vi "ChangeInheritance.vi"(0 "ClassWriterGOOP300 in":refnum<class "ClassWriterGOOP400.lvclass">, 1 "LvClass":refnum<vi>, 2 "NewBaseClass(Empty=ConvertClassToBaseClass)":path=path "C:/Documents and Settings/Micke/Skrivbord/My Computer/B_class/B.lvclass", 5 "error in (no error)":errorcluster) -> (14 "ClassWriterGOOP300 out":refnum<class "ClassWriterGOOP400.lvclass">, 19 "error out":errorcluster)   [LabVIEW 2020, in "ClassWriterGOOP400.lvclass"]
uses:
  <resource>/Framework/Providers/Open_GDS/ClassProviders/Provider_EndevoGOOP400/ClassWriterGOOP400_class/ClassWriterGOOP400.lvclass
  <resource>/Framework/Providers/Open_GDS/ClassProviders/Provider_EndevoGOOP400/Templates/EndevoG4TemplateNames.ctl
  <resource>/Framework/Providers/Open_GDS/ClassProviders/Provider_LvNativeClass/ClassWriterNative_class/ClassWriterNative.lvclass
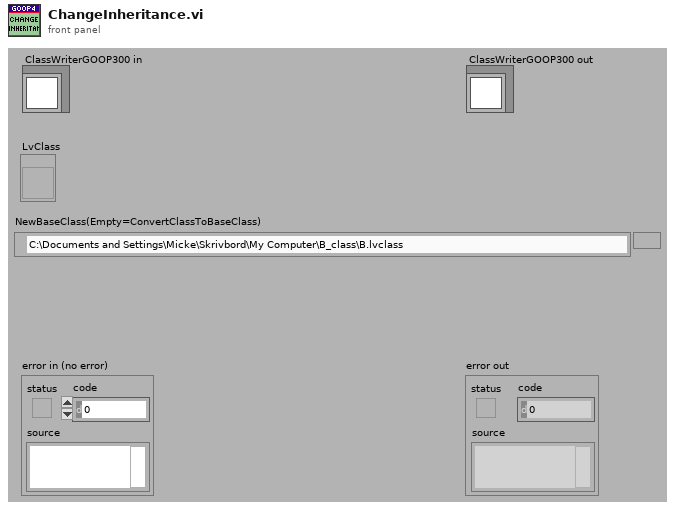
[diagram p1: front panel]
types:
  T1 = typedef "EndevoG4TemplateNames.ctl" = enum16{"G4BaseTemplate_Simple_4x4x4", "G4SubTemplate_Simple_4x4x4", "G4BaseTemplate_Simple_6x8x6", "G4SubTemplate_Simple_6x8x6", "G4BaseTemplate_Singleton_4x4x4", "G4SubTemplate_Singleton_4x4x4", "G4BaseTemplate_Singleton_6x8x6", "G4SubTemplate_Singleton_6x8x6", "G4InterfaceTemplate_6x8x6", "G4InterfaceTemplate_4x4x4", "G4BaseTemplate_Simple_5x6x5", "G4BaseTemplate_Singleton_5x6x5", "G4InterfaceTemplate_5x6x5", "G4SubTemplate_Simple_5x6x5", "G4SubTemplate_Singleton_5x6x5"}
  T2 = typedef "GDSLvCLass_ClassSettingsType.ctl" = cluster{"ClassProviderName":string, "ClassTemplateUsed":string, "ClassTemplateVersion":string, "ClassDescription":string, "PlugIns":T3[], "ConnectorPanePattern":string}
  T3 = typedef "GDSLvClass_PlugIn.ctl" = cluster{"Type":T4, "ID":string, "Version":string, "Path":path, "Name":string, "Data":variant}
  T4 = typedef "GDSLvClass_PlugInTypes.ctl" = enum16{"DesignPattern", "MethodTypes"}
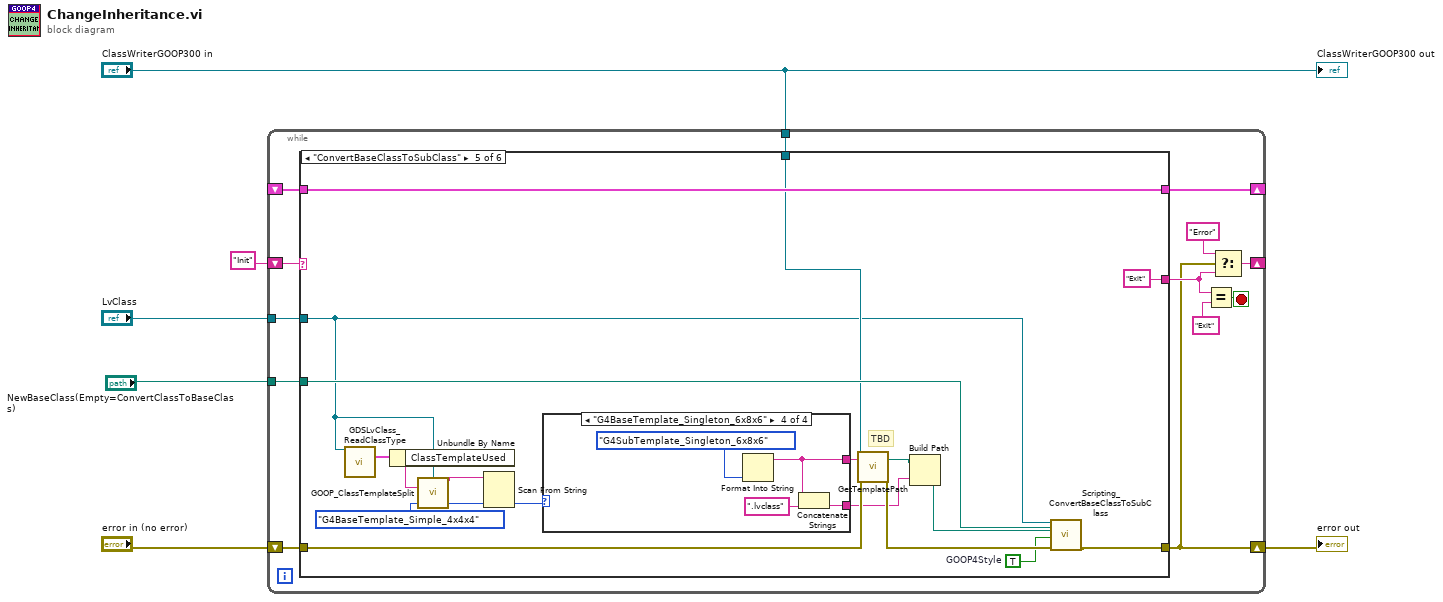
[diagram p0: block diagram]
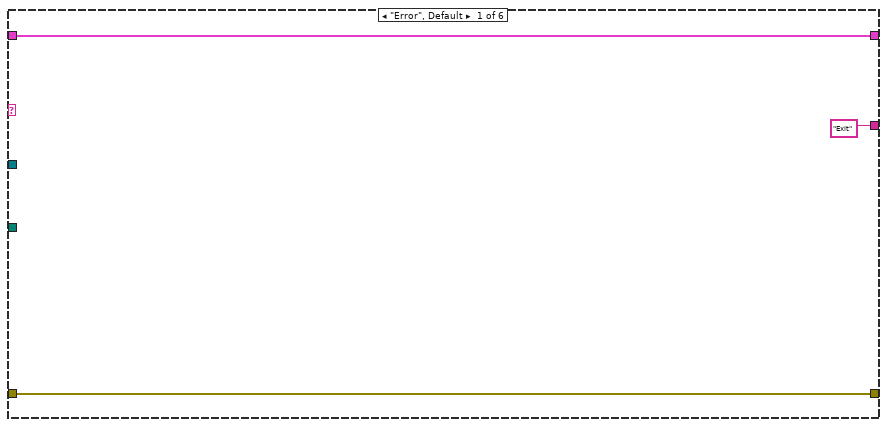
[diagram p2: hidden frame]
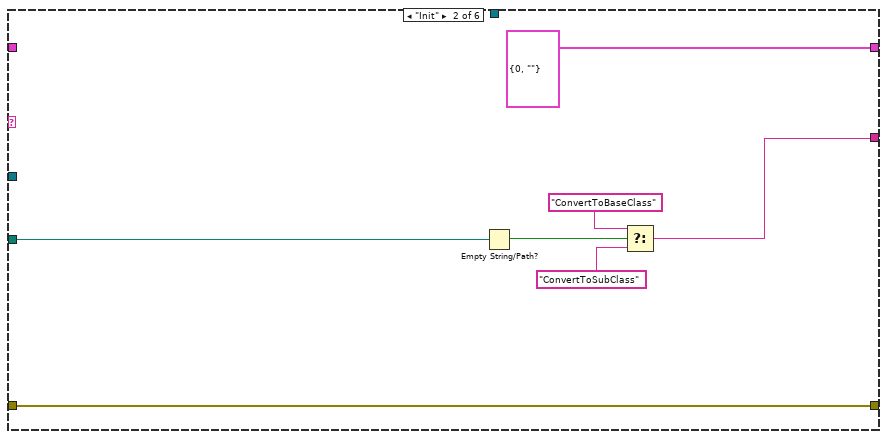
[diagram p3: hidden frame]
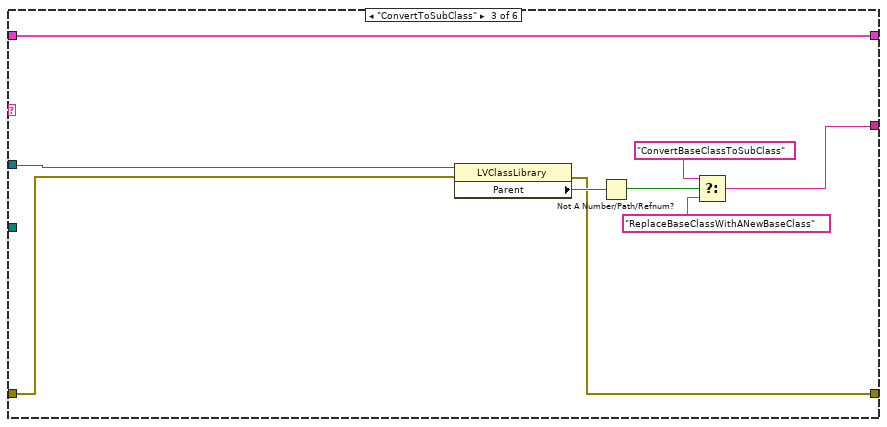
[diagram p4: hidden frame]
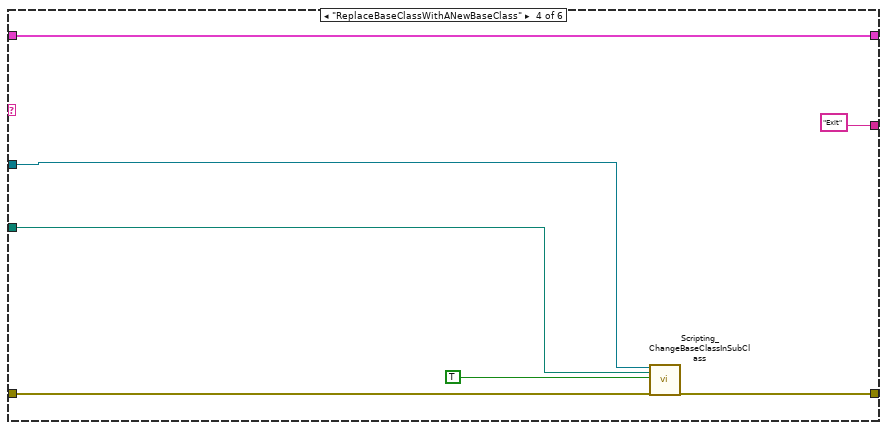
[diagram p5: hidden frame]
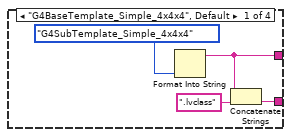
[diagram p6: hidden frame]
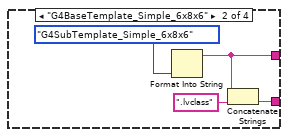
[diagram p7: hidden frame]
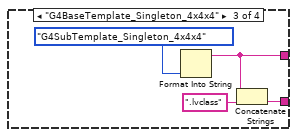
[diagram p8: hidden frame]
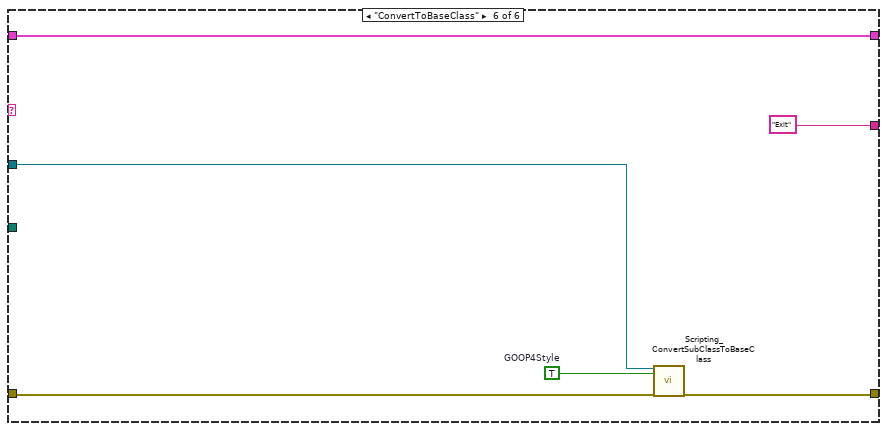
[diagram p9: hidden frame]
diagram:
  n1 = while {
    shift-right: [w13] -> w4
    shift-left: "error in (no error)" -> [w19]
    shift-right: [w17] -> _
    shift-left: "Init" -> [w18]
    shift-right: [w12] -> _
    shift-left: _ -> [w11]
    tunnel: "NewBaseClass(Empty=ConvertClassToBaseClass)" -> [w10]
    tunnel: "LvClass" -> [w9]
    tunnel: "ClassWriterGOOP300 in" -> [w7]
    stop <- w16 stop-if-true
    n2 = case shown="\"ConvertBaseClassToSubClass\"" w18 {
      tunnel: w19 -> [w22 w29 w37 w43 w61 w83]
      tunnel: [w22 w29 w32 w42 w63 w81] -> w13
      tunnel: ["Exit" w24 w33 "Exit" "Exit" "Exit"] -> w14
      tunnel: [w20 cluster{"Counter":i32, "Text":string} {"Counter"=0, "Text"=""} w30 w45 w55 w85] -> w12
      tunnel: w11 -> [w20 _ w30 w45 w55 w85]
      tunnel: w10 -> [_ w27 _ w40 w54 _]
      tunnel: w9 -> [_ _ w38 w41 w46 w82]
      tunnel: w7 -> [_ _ _ _ w53 _]
      frame "Error", Default {
      }
      frame "Init" {
        n3 = Empty String/Path?(string/path=w27) -> (empty?=w26:bool)
        n4 = Select(t="ConvertToBaseClass", s=w26, f="ConvertToSubClass") -> (s? t:f=w24:string)
      }
      frame "ConvertToSubClass" {
        n5 = property class="LVClassLibrary"(reference=w38, error in=w37) -> (error out=w32:errorcluster, "Parent"=w36:refnum<vi>)  [unwired: 1 out]
        n6 = Not A Number/Path/Refnum?(number/path/refnum=w36) -> (NaN/Path/Refnum?=w35:bool)
        n7 = Select(t="ConvertBaseClassToSubClass", s=w35, f="ReplaceBaseClassWithANewBaseClass") -> (s? t:f=w33:string)
      }
      frame "ReplaceBaseClassWithANewBaseClass" {
        n8 = call <resource>:"Scripting_ChangeBaseClassInSubClass.vi"("SubClass"=w41, "NewBaseClass"=w40, "GOOP4Style"=TRUE, "error in (no error)"=w43) -> ("error out"=w42:errorcluster)  [unwired: 15 in]
      }
      frame "ConvertBaseClassToSubClass" {
        w49 = TRUE  # GOOP4Style
        # "TBD"
        n9 = call <resource>:"GDSLvClass_ReadClassType.vi"("Class Refnum In"=w46) -> ("ClassSettings"=w52:T2)  [unwired: 16 in, 2 out]
        n10 = Unbundle By Name(w52) -> ("ClassTemplateUsed"=w47:string)
        n11 = call <resource>:"GOOP_ClassTemplateSplit.vi"("ClassItemRefIn"=w46, "FullClassTemplate"=w47) -> ("StandardTemplate"=w48:string)  [unwired: 12 in, 1 out]
        n12 = Scan From String(input string=w48, default 1=EndevoG4TemplateNames."G4BaseTemplate_Simple_4x4x4" ("TemplateNames")) -> (output 1=w50:T1)  [unwired: 3 in, 3 out]
        n13 = case shown="\"G4BaseTemplate_Singleton_6x8x6\"" w50 {
          tunnel: [w65 w69 w73 w77] -> w62
          tunnel: [w66 w70 w74 w78] -> w57
          frame "G4BaseTemplate_Simple_4x4x4", Default {
            n14 = Format Into String(EndevoG4TemplateNames."G4SubTemplate_Simple_4x4x4" ("TemplateNames")) -> (resulting string=w65:string)  [unwired: 3 in, 1 out]
            n15 = Concatenate Strings(w65, ".lvclass" ("name or relative path")) -> (w66:string)
          }
          frame "G4BaseTemplate_Simple_6x8x6" {
            n16 = Format Into String(EndevoG4TemplateNames."G4SubTemplate_Simple_6x8x6" ("TemplateNames")) -> (resulting string=w69:string)  [unwired: 3 in, 1 out]
            n17 = Concatenate Strings(w69, ".lvclass" ("name or relative path")) -> (w70:string)
          }
          frame "G4BaseTemplate_Singleton_4x4x4" {
            n18 = Format Into String(EndevoG4TemplateNames."G4SubTemplate_Singleton_4x4x4" ("TemplateNames")) -> (resulting string=w73:string)  [unwired: 3 in, 1 out]
            n19 = Concatenate Strings(w73, ".lvclass" ("name or relative path")) -> (w74:string)
          }
          frame "G4BaseTemplate_Singleton_6x8x6" {
            n20 = Format Into String(EndevoG4TemplateNames."G4SubTemplate_Singleton_6x8x6" ("TemplateNames")) -> (resulting string=w77:string)  [unwired: 3 in, 1 out]
            n21 = Concatenate Strings(w77, ".lvclass" ("name or relative path")) -> (w78:string)
          }
        }
        n22 = call-dynamic "GetTemplatePath.vi"("reference in"=w53, "ClassTemplateSubDirectory"=w62, "error in (no error)"=w61) -> ("FolderPathOut"=w59:path, "error out"=w60:errorcluster)  [unwired: 12 in, 3 out]
        n23 = Build Path(base path=w59, name or relative path=w57) -> (appended path=w58:path)
        n24 = call <resource>:"Scripting_ConvertBaseClassToSubClass.vi"("BaseClass"=w46, "NewBaseClass"=w54, "SubClassTemplate"=w58, "GOOP4Style"=w49, "error in (no error)"=w60) -> ("error out"=w63:errorcluster)  [unwired: 14 in]
      }
      frame "ConvertToBaseClass" {
        w80 = TRUE  # GOOP4Style
        n25 = call <resource>:"Scripting_ConvertSubClassToBaseClass.vi"("SubClass"=w82, "GOOP4Style"=w80, "error in (no error)"=w83) -> ("error out"=w81:errorcluster)  [unwired: 16 in]
      }
    }
    n26 = Equal?(x=w14, y="Exit") -> (x = y?=w16:bool)
    n27 = Select(t="Error", s=w13, f=w14) -> (s? t:f=w17:string)
  }
  "error out" <- w4
  "ClassWriterGOOP300 out" <- "ClassWriterGOOP300 in"
